vi "MQTT_PubRel_Read.vi"(8 "error in (no error)":errorcluster, 11 "connection ID":refnum<k5>) -> (0 "error out":errorcluster, 2 "Message ID":u16=10 format="%x", 3 "connection ID out":refnum<k5>)   [LabVIEW 2012, in "MQTT_Functions.lvlib"]
uses:
  MQTT_Functions.lvlib
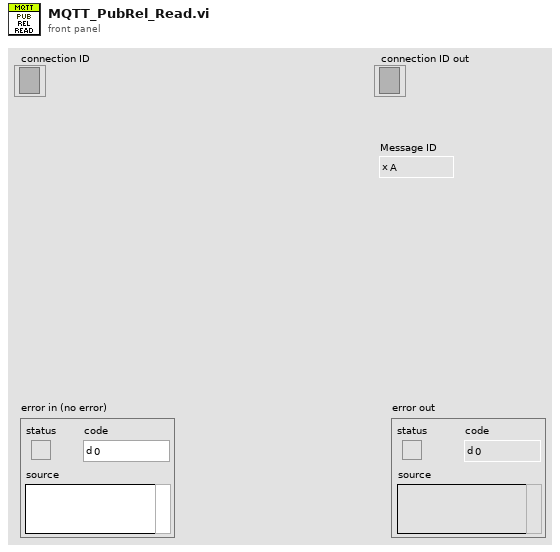
[diagram p1: front panel]
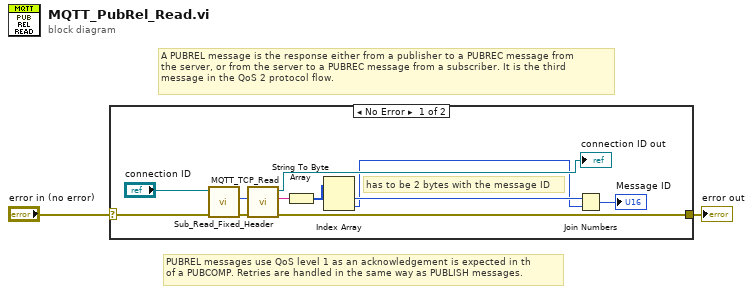
[diagram p0: block diagram]
diagram:
  # "PUBREL messages use QoS level 1 as an acknowledgement is expected in th\nof a PUBCOMP. Retries are handled in the same way as PUBLISH messages."
  # "A PUBREL message is the response either from a publisher to a PUBREC message from\nthe server, or from the server to a PUBREC message from a subscriber. It is the third\nmessage in the QoS 2 protocol flow."
  n1 = case shown="No Error" "error in (no error)" {
    selector: "error in (no error)" -> [w10 w14]
    tunnel: [w4 w14] -> w1
    frame No Error {
      # "has to be 2 bytes with the message ID"
      n2 = call "Sub_Read_Fixed_Header.vi"("error in (no error)"=w10, "connection ID"="connection ID") -> ("error out"=w5:errorcluster, "Remaining Length"=w11:u32)  [unwired: 3 in, 5 out]
      n3 = call "MQTT_TCP_Read.vi"("error in (no error)"=w5, "bytes to read"=w11) -> ("error out"=w4:errorcluster, "data out"=w6:string, "connection ID out"=→"connection ID out":refnum<k5>)  [unwired: 7 in]
      n4 = String To Byte Array(string=w6) -> (unsigned byte array=w7:u8[])
      n5 = Index Array(array=w7) -> (element #1=w9:u8, element #2=w8:u8)  [unwired: 2 in]
      n6 = Join Numbers(hi=w9, lo=w8) -> ((hi.lo)=→"Message ID":u16)
    }
    frame Error {
    }
  }
  "error out" <- w1
